vi "setVoltage.vi"(7 "chn":string, 8 "error in (no error)":errorcluster, 10 "voltage [V]":dbl, 11 "PsuNiPxi in":refnum<class "PsuNi.lvclass">) -> (0 "error out":errorcluster, 3 "PsuNiPxi out":refnum<class "PsuNi.lvclass">)   [LabVIEW 2023, in "PsuNi.lvclass"]
doc: "<b>Author:</b> Wolfgang\n<b>Description:</b> set output voltage of power supply by channel in V."
uses:
  PsuNi.lvclass
  PsuNi.lvclass/PsuNi.ctl
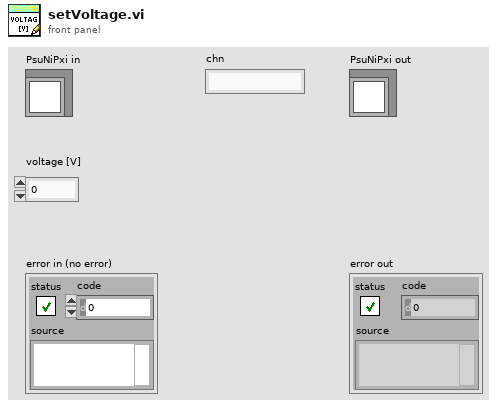
[diagram p1: front panel]
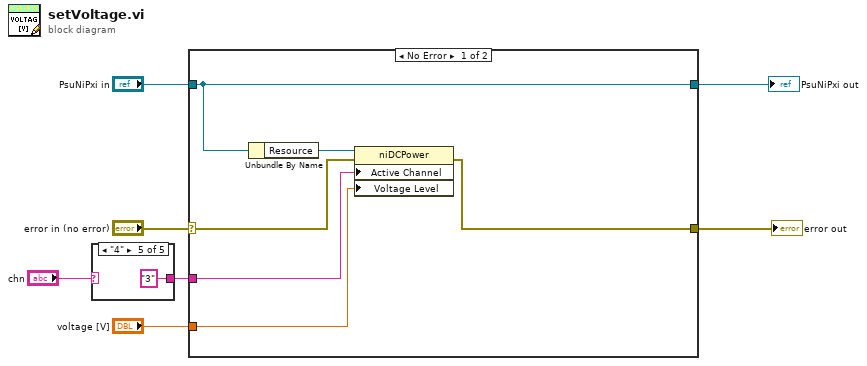
[diagram p0: block diagram]
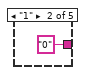
[diagram p3: hidden frame]
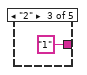
[diagram p4: hidden frame]
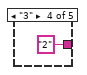
[diagram p5: hidden frame]
diagram:
  n1 = case shown="\"4\"" "chn" {
    selector: "chn" -> [w8 _ _ _ _]
    tunnel: [w8 "0" "1" "2" "3"] -> w1
    frame "False", Default {
    }
    frame "1" {
    }
    frame "2" {
    }
    frame "3" {
    }
    frame "4" {
    }
  }
  n2 = case shown="No Error" "error in (no error)" {
    selector: "error in (no error)" -> [w14 w19]
    tunnel: [w13 w19] -> w7
    tunnel: [w18 w20] -> w6
    tunnel: "PsuNiPxi in" -> [w18 w20]
    tunnel: w1 -> [w16 _]
    tunnel: "voltage [V]" -> [w15 _]
    frame No Error {
      n3 = Unbundle By Name(w18) -> ("Resource"=w17:refnum<k15>)
      n4 = property class="niDCPower"(reference=w17, error in=w14, "Active Channel"=w16, "Voltage Level"=w15) -> (error out=w13:errorcluster)  [unwired: 1 out]
    }
    frame Error {
    }
  }
  "error out" <- w7
  "PsuNiPxi out" <- w6
